vi "Close.vi"(8 "error in":errorcluster, 11 "Cluster.lvclass in":refnum<class "Cluster.lvclass">) -> (0 "error out":errorcluster)   [LabVIEW 2023, in "Cluster.lvclass"]
uses:
  Cluster.lvclass
  Cluster.lvclass/Cluster.ctl
  <vilib>/ADAS Replay HIL/AdasHilServices/AdasHilChannelServices.lvlib
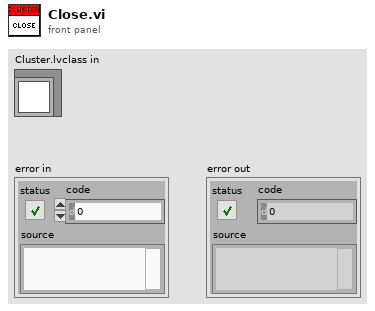
[diagram p1: front panel]
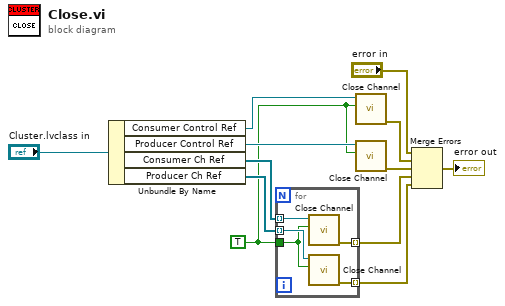
[diagram p0: block diagram]
diagram:
  w7 = TRUE ("Force Destroy? (F)")
  n1 = Unbundle By Name("Cluster.lvclass in") -> ("Consumer Control Ref"=w11:refnum<k21>, "Producer Control Ref"=w10:refnum<k21>, "Consumer Ch Ref"=w9:refnum<k21>[], "Producer Ch Ref"=w8:refnum<k21>[])
  n2 = for {
    tunnel: w9 -> [w17] mode=indexing
    tunnel: w8 -> [w16] mode=indexing
    tunnel: w7 -> [w15]
    tunnel: [w14] -> w1 mode=indexing
    tunnel: [w13] -> w2 mode=indexing
    n3 = call <vilib>:"Close Channel.vi"("Force Destroy? (F)"=w15, "ADAS HIL Channel"=w17) -> ("error out"=w13:errorcluster)  [unwired: 9 in]
    n4 = call <vilib>:"Close Channel.vi"("Force Destroy? (F)"=w15, "ADAS HIL Channel"=w16) -> ("error out"=w14:errorcluster)  [unwired: 9 in]
  }
  n5 = call <vilib>:"Close Channel.vi"("Force Destroy? (F)"=w7, "ADAS HIL Channel"=w11) -> ("error out"=w4:errorcluster)  [unwired: 9 in]
  n6 = call <vilib>:"Close Channel.vi"("Force Destroy? (F)"=w7, "ADAS HIL Channel"=w10) -> ("error out"=w3:errorcluster)  [unwired: 9 in]
  n7 = Merge Errors("error in", w4, w3, w2, w1) -> (→"error out":errorcluster)
